vi "getCurrentCameras.vi"(4 "Camera 3":refnum<data-value>, 5 "Camera 0":refnum<data-value>, 6 "Camera 2":refnum<data-value>, 7 "Camera 1":refnum<data-value>, 8 "error in (no error)":errorcluster, 9 "Field Size":refnum<data-value>, 11 "Vision in":refnum<class "Vision.lvclass">) -> (0 "error out":errorcluster, 1 "Field Size out":T1, 2 "NewCameras":T2[](array[typedef]) {"robots_blue"."height" format="%+4.3f"; "robots_blue"."pixel_y" format="%+4.3f"; "robots_blue"."pixel_x" format="%+4.3f"; "robots_blue"."orientation" format="%+4.3f"; "robots_blue"."y" format="%+4.3f"; "robots_blue"."confidence" format="%4.3f"; "robots_blue"."x" format="%+4.3f"; "robots_yellow"."height" format="%+4.3f"; "robots_yellow"."pixel_y" format="%+4.3f"; "robots_yellow"."pixel_x" format="%+4.3f"; "robots_yellow"."orientation" format="%+4.3f"; "robots_yellow"."y" format="%+4.3f"; "robots_yellow"."confidence" format="%4.3f"; "robots_yellow"."x" format="%+4.3f"}, 3 "Vision out":refnum<class "Vision.lvclass">)   [LabVIEW 2023, in "Vision.lvclass"]
uses:
  Vision.lvclass
  Old vision/Controls/SSL Detection Frame.ctl
  Old vision/Controls/SSL Detection Robot.ctl
  <vilib>/Analysis/Matrix/Datatypes/RealMatrix.ctl
  Old vision/Controls/SSL Detection Ball.ctl
  <vilib>/Analysis/Matrix/NI_Matrix.lvlib
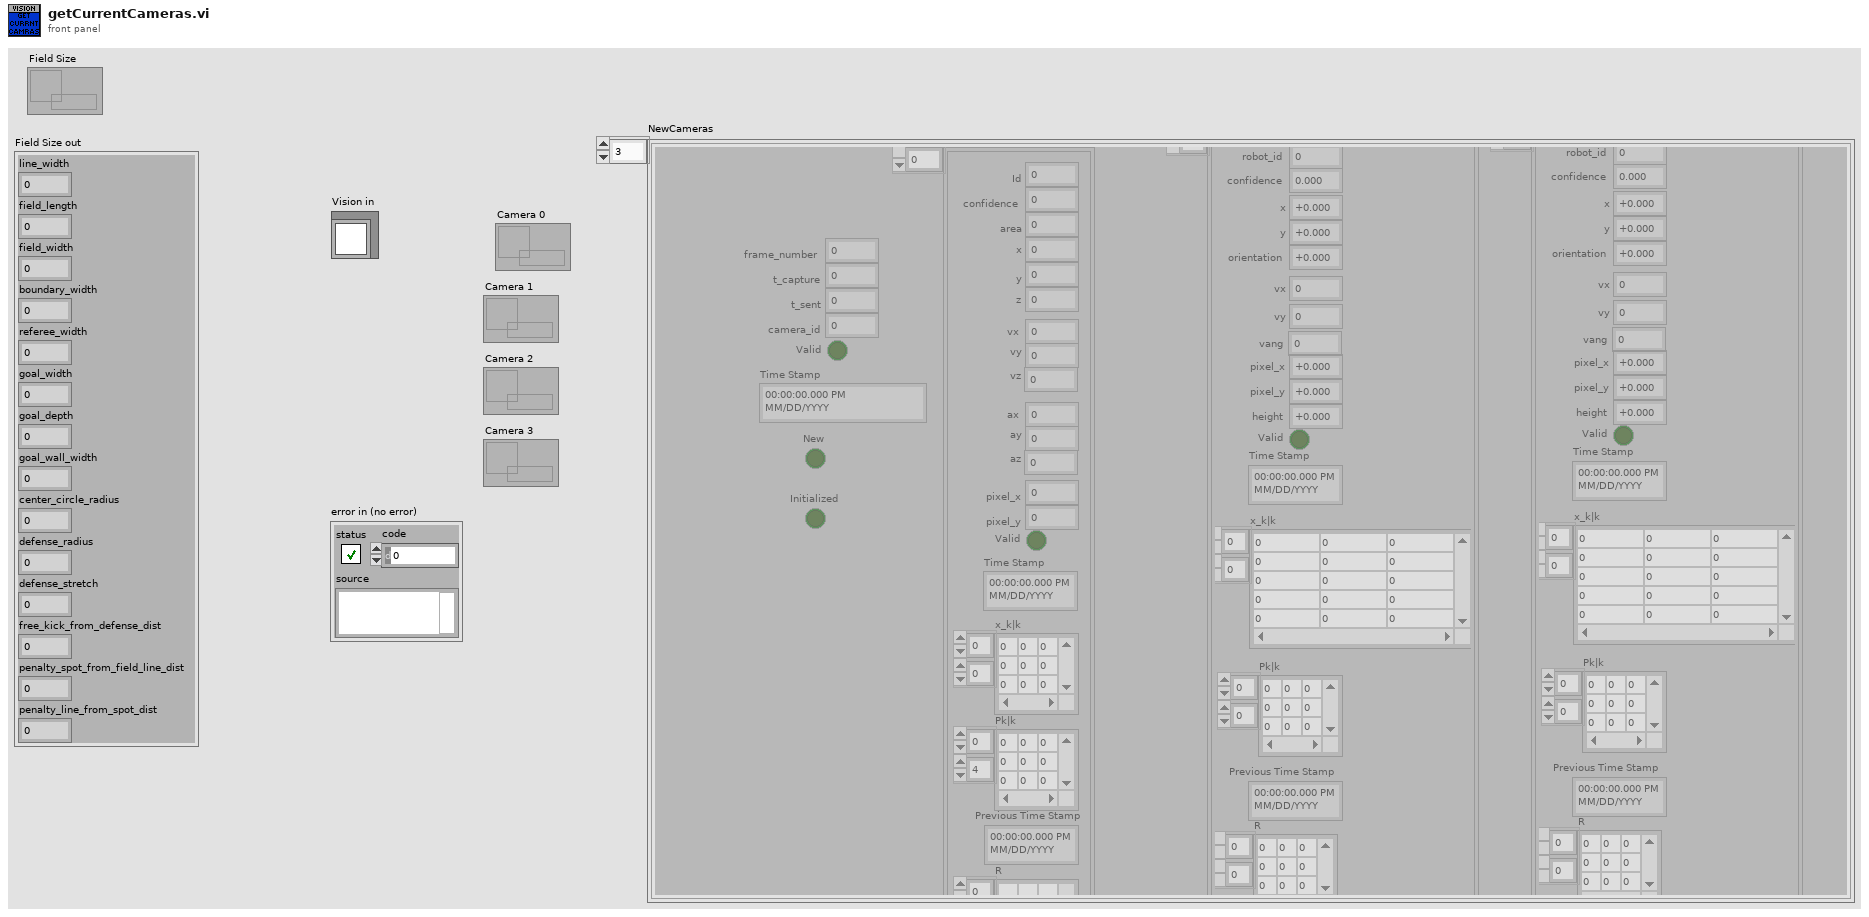
[diagram p1: front panel]
types:
  T1 = cluster{"line_width":u32, "field_length":u32, "field_width":u32, "boundary_width":u32, "referee_width":u32, "goal_width":u32, "goal_depth":u32, "goal_wall_width":u32, "center_circle_radius":u32, "defense_radius":u32, "defense_stretch":u32, "free_kick_from_defense_dist":u32, "penalty_spot_from_field_line_dist":u32, "penalty_line_from_spot_dist":u32}
  T2 = typedef "SSL Detection Frame.ctl" = cluster{"frame_number":u32, "t_capture":dbl, "t_sent":dbl, "camera_id":u32, "robots_yellow":T3[], "robots_blue":T3[], "balls":T5[], "Valid":bool, "Time Stamp":timestamp, "New":bool, "Initialized":bool}
  T3 = typedef "SSL Detection Robot.ctl" = cluster{"x":sgl, "robot_id":u32, "confidence":sgl, "y":sgl, "orientation":sgl, "pixel_x":sgl, "pixel_y":sgl, "height":sgl, "Valid":bool, "Time Stamp":timestamp, "x_k|k":T4, "Pk|k":T4, "Previous Time Stamp":timestamp, "R":T4, "vx":dbl, "vy":dbl, "vang":dbl}
  T4 = typedef "NI_Matrix.lvlib/RealMatrix.ctl" = dbl[][]
  T5 = typedef "SSL Detection Ball.ctl" = cluster{"x":sgl, "area":u32, "confidence":sgl, "y":sgl, "z":sgl, "pixel_x":sgl, "pixel_y":sgl, "Valid":bool, "Time Stamp":timestamp, "x_k|k":T4, "Pk|k":T4, "Id":u32, "Previous Time Stamp":timestamp, "R":T4, " vx":sgl, "vy":dbl, "vz":dbl, " ax":sgl, "ay":dbl, "az":dbl}
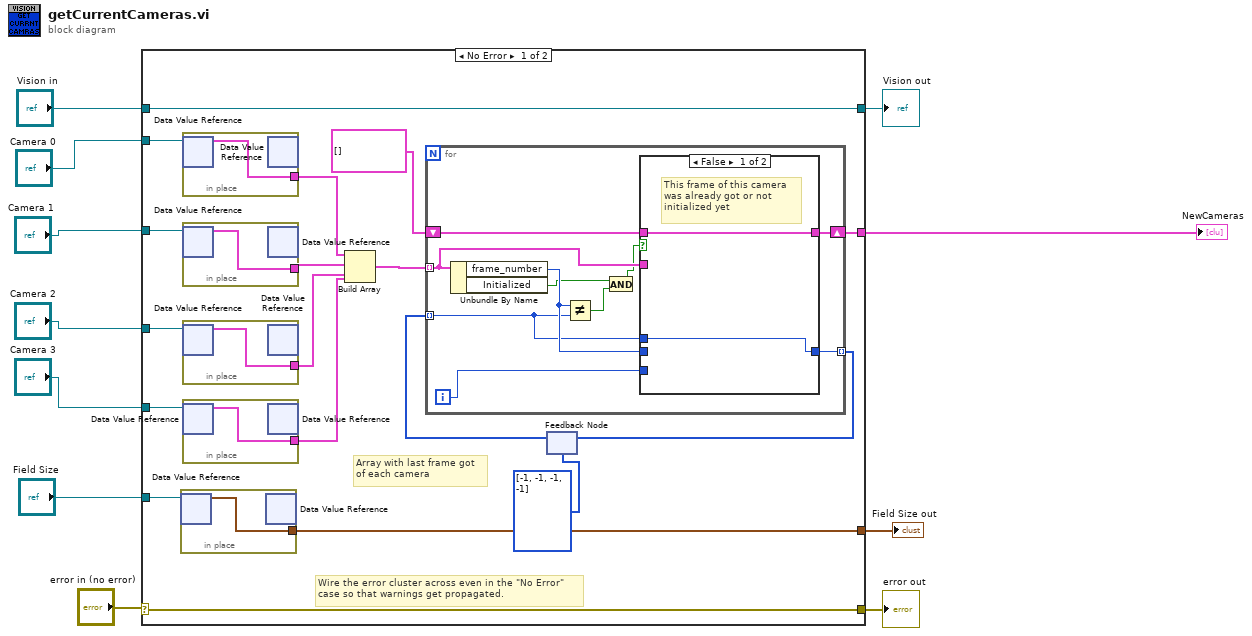
[diagram p0: block diagram]
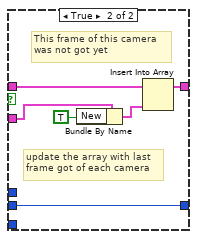
[diagram p2: hidden frame]
diagram:
  n1 = case shown="No Error" "error in (no error)" {
    selector: "error in (no error)" -> [w28 w54]
    tunnel: [w28 w54] -> w10
    tunnel: [w29 w53] -> w8
    tunnel: "Vision in" -> [w29 w53]
    tunnel: "Camera 0" -> [w27 _]
    tunnel: "Camera 1" -> [w26 _]
    tunnel: "Camera 2" -> [w24 _]
    tunnel: "Camera 3" -> [w25 _]
    tunnel: [w17 _] -> w1
    tunnel: "Field Size" -> [w13 _]
    tunnel: [w12 _] -> w2
    frame No Error {
      # "Array with last frame got\nof each camera"
      # "Wire the error cluster across even in the \"No Error\"\ncase so that warnings get propagated."
      n2 = in-place {
        in-place-border: [w30] -> w12
        n3 = in-place-dvr #1(w13) -> (w30:T1)  [unwired: 1 out]
        n4 = in-place-dvr #1() -> ()  [unwired: 1 in, 2 out]
      }
      n5 = in-place {
        in-place-border: [w52] -> w23
        n6 = in-place-dvr #2(w27) -> (w52:T2)  [unwired: 1 out]
        n7 = in-place-dvr #2() -> ()  [unwired: 1 in, 2 out]
      }
      n8 = in-place {
        in-place-border: [w51] -> w22
        n9 = in-place-dvr #3(w26) -> (w51:T2)  [unwired: 1 out]
        n10 = in-place-dvr #3() -> ()  [unwired: 1 in, 2 out]
      }
      n11 = in-place {
        in-place-border: [w50] -> w21
        n12 = in-place-dvr #4(w24) -> (w50:T2)  [unwired: 1 out]
        n13 = in-place-dvr #4() -> ()  [unwired: 1 in, 2 out]
      }
      n14 = in-place {
        in-place-border: [w49] -> w20
        n15 = in-place-dvr #5(w25) -> (w49:T2)  [unwired: 1 out]
        n16 = in-place-dvr #5() -> ()  [unwired: 1 in, 2 out]
      }
      n17 = Build Array(w23, w22, w21, w20) -> (w19:T2[])
      n18 = feedback #6(i32[] [-1, -1, -1, -1] ("frame_number")) -> (w15:u32[])
      n19 = for {
        tunnel: w19 -> [w40] mode=indexing
        shift-right: [w38] -> w17
        shift-left: T2[] [] ("NewCameras 2") -> [w39]
        tunnel: w15 -> [w34] mode=indexing
        tunnel: [w36] -> w14 mode=indexing
        i -> [w37]
        n20 = Unbundle By Name(w40) -> ("frame_number"=w35:u32, "Initialized"=w32:bool)
        n21 = Not Equal?(x=w35, y=w34) -> (x != y?=w33:bool)
        n22 = And(x=w32, y=w33) -> (x .and. y?=w31:bool)
        n23 = case shown="False" w31 {
          tunnel: w40 -> [_ w45]
          tunnel: w39 -> [w42 w48]
          tunnel: [w42 w47] -> w38
          tunnel: w37 -> [_ _]
          tunnel: [w41 w46] -> w36
          tunnel: w35 -> [_ w46]
          tunnel: w34 -> [w41 _]
          frame False {
            # "This frame of this camera \nwas already got or not\ninitialized yet"
          }
          frame True {
            # "update the array with last\nframe got of each camera"
            # "This frame of this camera \nwas not got yet"
            n24 = Bundle By Name(cluster=w45, "New"=TRUE) -> (w44:T2)
            n25 = Insert Into Array(array=w48, new element=w44) -> (w47:T2[])  [unwired: 1 in]
          }
        }
      }
      n26 = feedback-in #6(w14) -> ()
    }
    frame Error {
    }
  }
  "error out" <- w10
  "Vision out" <- w8
  "NewCameras" <- w1
  "Field Size out" <- w2
